vi "initialise_main.vi"(8 "error in (no error)":errorcluster, 11 "control references in":T3) -> (0 "error out":errorcluster, 3 "configuration":T1)   [LabVIEW 2010]
uses:
  common/classes/GenericComponent/GenericComponent/GenericComponent.lvclass
  global_variables.vi
  components/Stage/GenericStage/GenericStage/GenericStage.lvclass
  common/classes/NoteBook/Notebook/Notebook.lvclass
  components/Objective/GenericObjective/GenericObjective/GenericObjective.lvclass
  common/xcontrols/XUserDropdown/XUserDropdown/XUserDropdown.xctl
  type_definitions/clusters/controls_refs.ctl
  common/clusters/plugin_specification.ctl
  type_definitions/clusters/top_level_config_cluster.ctl
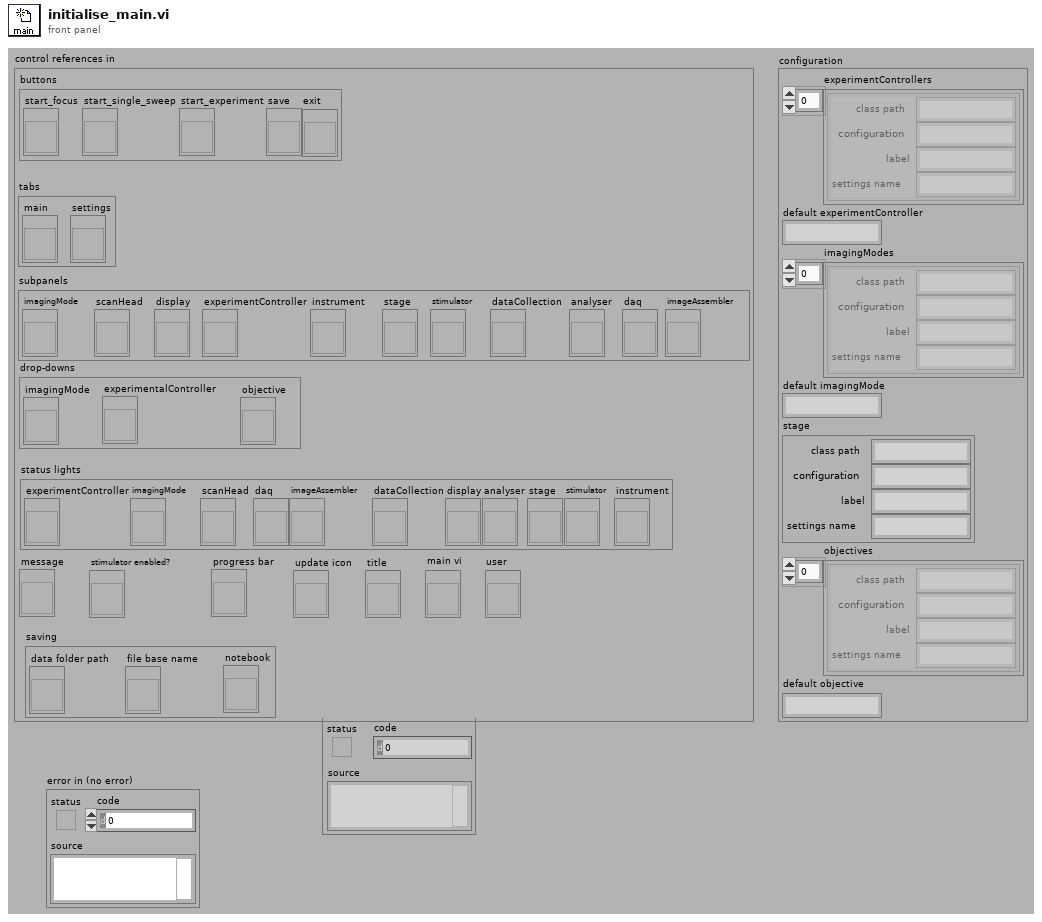
[diagram p1: front panel]
types:
  T1 = typedef "top_level_config_cluster.ctl" = cluster{"experimentControllers":T2[], "default experimentController":string, "imagingModes":T2[], "default imagingMode":string, "stage":T2, "objectives":T2[], "default objective":string}
  T2 = typedef "plugin_specification.ctl" = cluster{"class path":string, "configuration":string, "label":string, "settings name":string}
  T3 = typedef "controls_refs.ctl" = cluster{"buttons":cluster{"start_focus":refnum<vi>, "start_single_sweep":refnum<vi>, "start_experiment":refnum<vi>, "save":refnum<vi>, "exit":refnum<vi>}, "tabs":cluster{"main":refnum<vi>, "settings":refnum<vi>}, "subpanels":cluster{"imagingMode":refnum<vi>, "scanHead":refnum<vi>, "display":refnum<vi>, "experimentController":refnum<vi>, "instrument":refnum<vi>, "stage":refnum<vi>, "stimulator":refnum<vi>, "dataCollection":refnum<vi>, "analyser":refnum<vi>, "daq":refnum<vi>, "imageAssembler":refnum<vi>}, "drop-downs":cluster{"imagingMode":refnum<vi>, "experimentalController":refnum<vi>, "objective":refnum<vi>}, "status lights":cluster{"experimentController":refnum<vi>, "imagingMode":refnum<vi>, "scanHead":refnum<vi>, "daq":refnum<vi>, "imageAssembler":refnum<vi>, "dataCollection":refnum<vi>, "display":refnum<vi>, "analyser":refnum<vi>, "stage":refnum<vi>, "stimulator":refnum<vi>, "instrument":refnum<vi>}, "message":refnum<vi>, "stimulator enabled?":refnum<vi>, "saving":cluster{"data folder path":refnum<vi>, "file base name":refnum<vi>, "notebook":refnum<vi>}, "progress bar":refnum<vi>, "update icon":refnum<vi>, "title":refnum<vi>, "main vi":refnum<vi>, "user":refnum<vi>}
  T4 = cluster{"experimentController":refnum<vi>, "imagingMode":refnum<vi>, "scanHead":refnum<vi>, "daq":refnum<vi>, "imageAssembler":refnum<vi>, "dataCollection":refnum<vi>, "display":refnum<vi>, "analyser":refnum<vi>, "stage":refnum<vi>, "stimulator":refnum<vi>, "instrument":refnum<vi>}
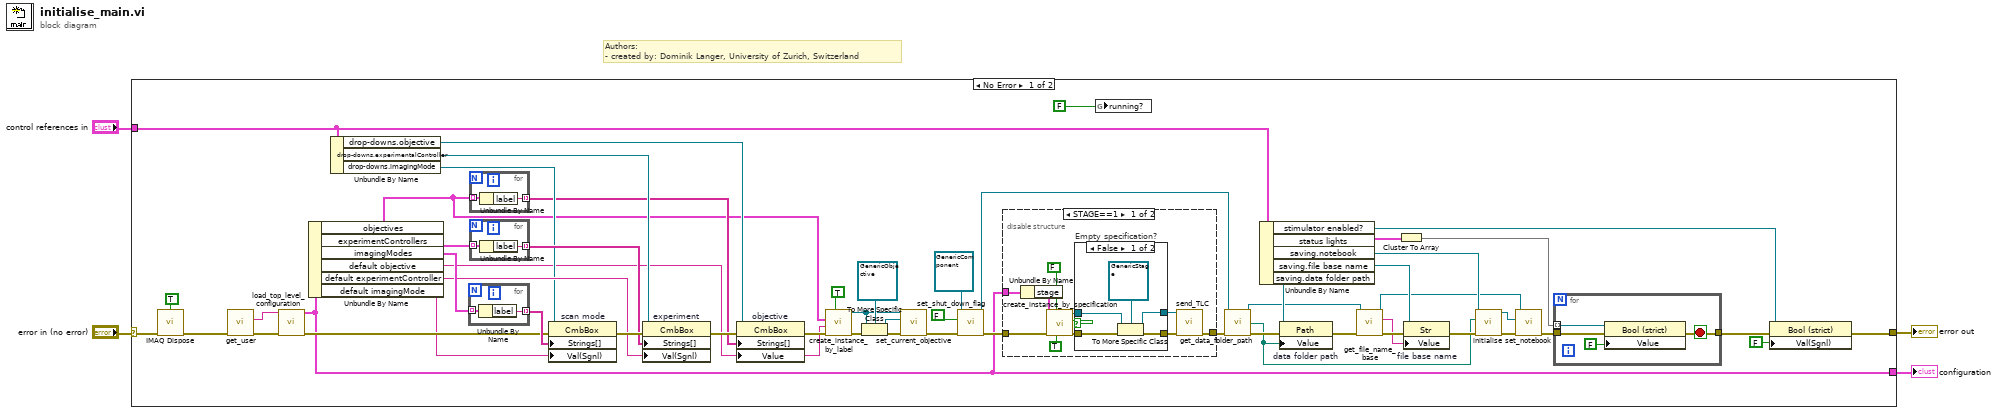
[diagram p0: block diagram]
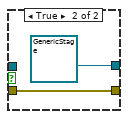
[diagram p2: hidden frame]
diagram:
  # "Authors: \n- created by: Dominik Langer, University of Zurich, Switzerland"
  n1 = case shown="No Error" "error in (no error)" {
    selector: "error in (no error)" -> [w11 w90]
    tunnel: [w6 w90] -> w4
    tunnel: [w35 _] -> w2
    tunnel: "control references in" -> [w32 _]
    frame No Error {
      n2 = call "IMAQ Dispose"("All Images? (No)"=TRUE, "error in (no error)"=w11) -> ("error out"=w10:errorcluster)  [unwired: 4 in]
      n3 = call "get_user.vi"("error in (no error)"=w10) -> ("error out"=w16:errorcluster, "username out"=w17:string)  [unwired: 9 in]
      n4 = call "load_top_level_configuration.vi"("error in (no error)"=w16, "user"=w17) -> ("error out"=w58:errorcluster, "configuration"=w35:T1)  [unwired: 2 in, 6 out]
      n5 = Unbundle By Name(w35) -> ("objectives"=w38:T2[], "experimentControllers"=w56:T2[], "imagingModes"=w57:T2[], "default objective"=w39:string, "default experimentController"=w54:string, "default imagingMode"=w55:string)
      n6 = Unbundle By Name(w32) -> ("drop-downs.objective"=w48:refnum<vi>, "drop-downs.experimentalController"=w52:refnum<vi>, "drop-downs.imagingMode"=w51:refnum<vi>)
      n7 = for {
        tunnel: w57 -> [w87] mode=indexing
        tunnel: [w86] -> w60 mode=indexing
        n8 = Unbundle By Name(w87) -> ("label"=w86:string)
      }
      n9 = for {
        tunnel: w38 -> [w85] mode=indexing
        tunnel: [w84] -> w47 mode=indexing
        n10 = Unbundle By Name(w85) -> ("label"=w84:string)
      }
      n11 = for {
        tunnel: w56 -> [w89] mode=indexing
        tunnel: [w88] -> w53 mode=indexing
        n12 = Unbundle By Name(w89) -> ("label"=w88:string)
      }
      n13 = property on="scan mode" class="CmbBox"(reference=w51, error in=w58, "Strings[]"=w60, "Val(Sgnl)"=w55) -> (error out=w59:errorcluster)  [unwired: 1 out]
      n14 = property on="experiment" class="CmbBox"(reference=w52, error in=w59, "Strings[]"=w53, "Val(Sgnl)"=w54) -> (error out=w49:errorcluster)  [unwired: 1 out]
      n15 = property on="objective" class="CmbBox"(reference=w48, error in=w49, "Strings[]"=w47, "Value"=w39) -> (error out=w40:errorcluster)  [unwired: 1 out]
      n16 = call "create_instance_by_label.vi"("call constructor?"=TRUE, "error in (no error)"=w40, "label"=w39, "configuration list"=w38) -> ("error out"=w43:errorcluster, "GenericPlugin out"=w45:refnum<class "GenericComponent.lvclass">)  [unwired: 6 out]
      n17 = To More Specific Class(target class=refnum<class "GenericObjective.lvclass"> refnum ("GenericObjective.lvclass"), reference=w45, error in=w43) -> (specific class reference=w44:refnum<class "GenericObjective.lvclass">, error out=w42:errorcluster)
      n18 = call-dynamic "set_current_objective.vi"("error in (no error)"=w42, "current objective"=w44, "GenericPlugin in"=w45) -> ("error out"=w41:errorcluster)  [unwired: 7 in, 1 out]
      n19 = call-dynamic "set_shut_down_flag.vi"("error in (no error)"=w41, "shut down?"=FALSE, "GenericPlugin in"=refnum<class "GenericComponent.lvclass"> refnum ("GenericPlugin.lvclass")) -> ("error out"=w36:errorcluster, "GenericPlugin out"=w29:refnum<class "GenericComponent.lvclass">)  [unwired: 7 out]
      n20 = disable-structure shown="STAGE==1" {
        disable-tunnel: w36 -> [w74 w83]
        disable-tunnel: [w67 w83] -> w33
        disable-tunnel: w35 -> [w75 _]
        frame condition #0 (active) {
          n21 = Unbundle By Name(w75) -> ("stage"=w72:T2)
          n22 = call "create_instance_by_specification.vi"("be tolerant against empty specification?"=TRUE, "call constructor?"=FALSE, "error in (no error)"=w74, "component specification"=w72) -> ("error out"=w73:errorcluster, "empty specification!"=w71:bool, "GenericPlugin out"=w70:refnum<class "GenericComponent.lvclass">)  [unwired: 5 in]
          n23 = case "Empty specification?" shown="False" w71 {
            tunnel: [w77 w82] -> w66
            tunnel: w73 -> [w80 w82]
            tunnel: w70 -> [w78 _]
            tunnel: [w76 refnum<class "GenericStage.lvclass"> refnum ("GenericStage.lvclass")] -> w65
            frame False {
              n24 = To More Specific Class(target class=refnum<class "GenericStage.lvclass"> refnum ("GenericStage.lvclass"), reference=w78, error in=w80) -> (specific class reference=w76:refnum<class "GenericStage.lvclass">, error out=w77:errorcluster)
            }
            frame True {
            }
          }
          n25 = call-dynamic "send_TLC.vi"("error in (no error)"=w66, "GenericToplevelComponent in"=w65) -> ("error out"=w67:errorcluster)  [unwired: 8 in, 1 out]
        }
        frame condition #1 {
        }
      }
      n26 = global write "global_variables.vi" "running?"(FALSE) -> ()
      n27 = call-dynamic "get_data_folder_path.vi"("error in (no error)"=w33, "GenericComponent in"=w29) -> ("error out"=w27:errorcluster, "data folder path"=w21:path, "GenericComponent out"=w26:refnum<class "GenericComponent.lvclass">)  [unwired: 7 in]
      n28 = Unbundle By Name(w32) -> ("stimulator enabled?"=w8:refnum<vi>, "status lights"=w13:T4, "saving.notebook"=w22:refnum<vi>, "saving.file base name"=w28:refnum<vi>, "saving.data folder path"=w31:refnum<vi>)
      n29 = property on="data folder path" class="Path"(reference=w31, error in=w27, "Value"=w21) -> (error out=w30:errorcluster)  [unwired: 1 out]
      n30 = call-dynamic "get_file_name_base.vi"("error in (no error)"=w30, "GenericComponent in"=w26) -> ("error out"=w25:errorcluster, "file name base"=w24:string, "GenericComponent out"=w20:refnum<class "GenericComponent.lvclass">)  [unwired: 7 in]
      n31 = Cluster To Array(cluster=w13) -> (array=w14:refnum<vi>[])
      n32 = property on="file base name" class="Str"(reference=w28, error in=w25, "Value"=w24) -> (error out=w23:errorcluster)  [unwired: 1 out]
      n33 = call "initialise.vi"("error in (no error)"=w23, "folder path"=w21, "notebook control ref"=w22) -> ("error out"=w18:errorcluster, "Notebook out"=w19:refnum<class "Notebook.lvclass">)  [unwired: 7 out]
      n34 = call-dynamic "set_notebook.vi"("error in (no error)"=w18, "notebook"=w19, "GenericComponent in"=w20) -> ("error out"=w15:errorcluster)  [unwired: 7 in, 1 out]
      n35 = for {
        tunnel: w15 -> [w64]
        tunnel: [w62] -> w5
        tunnel: w14 -> [w63] mode=indexing
        stop <- w62 stop-if-true
        n36 = property class="Bool (strict)"(reference=w63, error in=w64, "Value"=FALSE) -> (error out=w62:errorcluster)  [unwired: 1 out]
      }
      n37 = property on="Property Node" class="Bool (strict)"(reference=w8, error in=w5, "Val(Sgnl)"=FALSE ("Value (Signaling)")) -> (error out=w6:errorcluster)  [unwired: 1 out]
    }
    frame Error {
    }
  }
  "error out" <- w4
  "configuration" <- w2
